vi "Stop Generation.vi"(0 "fpga interface in":refnum<k20>, 5 "stop timeout (s)":dbl=5.0 format="%#_13g", 11 "error in (no error)":errorcluster) -> (4 "fpga interface out":refnum<k20>, 15 "error out":errorcluster)   [LabVIEW 2023, in "GettingStarted_Gen_148X_Host.lvlib"]
uses:
  GettingStarted_Gen_148X_Host.lvlib
  Types/148x_Gen_FPGA_Reference.ctl
  <instrlib>/FlexRIO/CSI-2/v2/FPGA/Types/Generation Engine State.ctl
  <vilib>/Utility/error.llb/Error Cluster From Error Code.vi
  <vilib>/rvi/errors/niLvFpgaAdjustHostInterfaceError.vi
  <vilib>/rvi/interface/nirviReadWriteControl/nirviReadWriteControl.xnode
  <instrlib>/FlexRIO/CSI-2/v2/FPGA/NI CSI-2 API FPGA v2.lvlib
  NiFpgaLv.dll
  <vilib>/rvi/interface/Simulation/niFpgaSimulationCallBeginRW.vi
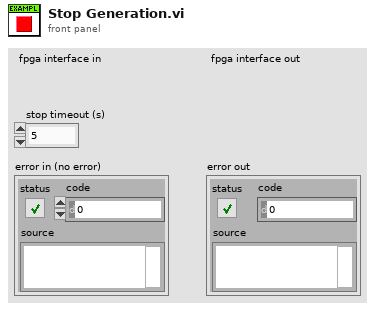
[diagram p1: front panel]
types:
  T1 = typedef "NI CSI-2 API FPGA v2.lvlib/Generation Engine State.ctl" = enum8{"Idle", "Ready For Start Trigger", "Generate Packets", "Done", "Error"}
  T2 = typedef "GettingStarted_Gen_148X_Host.lvlib/148x_Gen_FPGA_Reference.ctl" = refnum<k20>
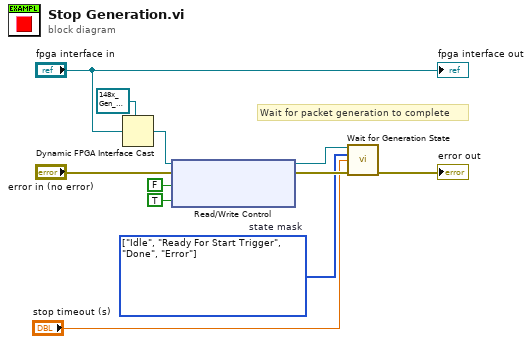
[diagram p0: block diagram]
diagram:
  w2 = T1[] [enum."Idle", enum."Ready For Start Trigger", enum."Done", enum."Error"] items=["Idle", "Ready For Start Trigger", "Generate Packets", "Done", "Error"]  # state mask
  # "Wait for packet generation to complete"
  n1 = Dynamic FPGA Interface Cast(Session In=T2 refnum ("FPGA VI Reference Out"), Type="fpga interface in") -> (Session Out=w7:T2)
  n2 = xnode "Read/Write Control"("FPGA VI Reference In"=w7, "error in"="error in (no error)", "sw start trigger"=FALSE ("stop trigger"), "stop trigger (strobe)"=TRUE) -> ("FPGA VI Reference Out"=w3:T2, "error out"=w5:errorcluster)
  n3 = call "Wait for Generation State.vi"("fpga interface in"=w3, "state mask"=w2, "timeout (s)"="stop timeout (s)", "error in (no error)"=w5) -> ("error out"=→"error out":errorcluster)  [unwired: 8 in, 3 out]
  "fpga interface out" <- "fpga interface in"
